vi "Find Workspace.vi"(6 "Pickup_Test_Number":dbl, 7 "Database Entry in":refnum<class "Database Entry.lvclass">, 8 "Error In":errorcluster, 9 "Assembly Type":string, 10 "Control In":T2={"I-O.lvclass"=refnum, "Gantry"=refnum, "Dispenser"="COM1"}, 11 "Workspace In":refnum<class "Fixture.lvclass">) -> (0 "Error Out":errorcluster, 1 "Workspace Out":T1, 2 "Control Out":T2={"I-O.lvclass"=refnum, "Gantry"=refnum, "Dispenser"="COM1"}, 3 "Workspace Out":refnum<class "Fixture.lvclass">, 5 "Database Entry out":refnum<class "Database Entry.lvclass">)   [LabVIEW 2021, in "Fixture.lvclass"]
uses:
  Fixture.lvclass
  Controller/Controllers.ctl
  Controller/I-O/I-O.lvclass
  C:/Program Files (x86)/Aerotech/A3200/LabVIEW/2010/Bin/Aerotech.A3200.dll
  Program Files (x86)/Aerotech/A3200/LabVIEW/2010/Bin/Aerotech.A3200.dll
  Workspace.ctl
  Assembly/Database Entry/Database Entry.lvclass
  Fixture.lvclass/Fixture.ctl
  Controller/Controller.lvclass
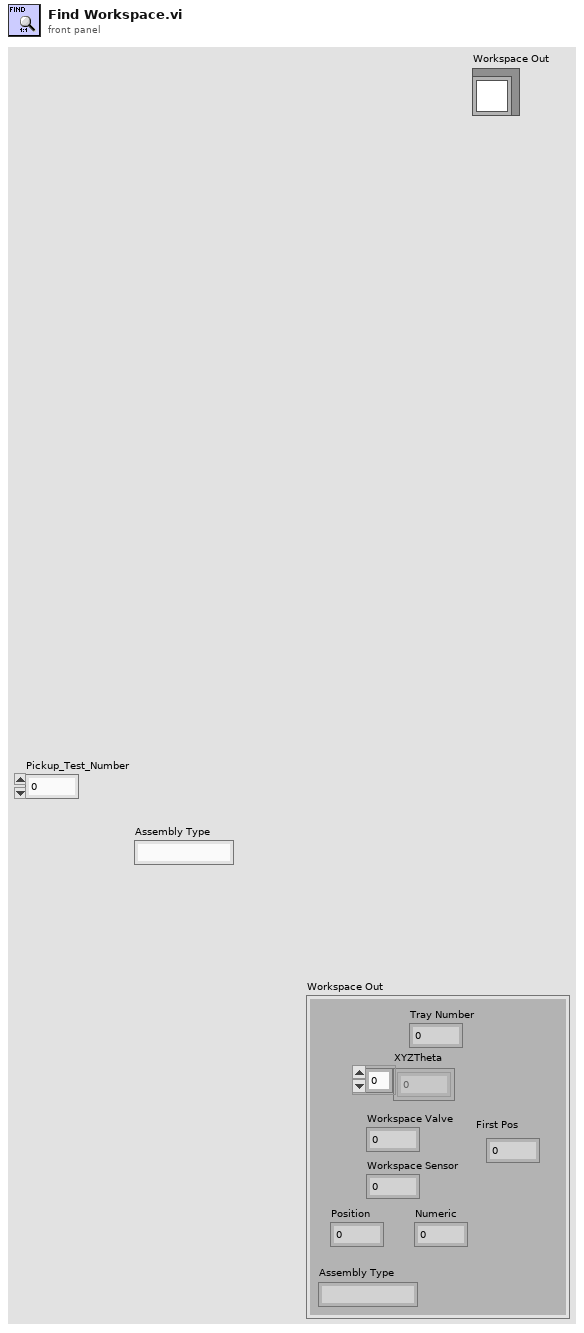
[diagram p1: front panel]
types:
  T1 = typedef "Fixture.lvclass/Workspace.ctl" = cluster{"XYZTheta":dbl[], "Workspace Valve":i32, "Workspace Sensor":i32, "Tray Number":i32, "Position":i32, "Assembly Type":string, "Numeric":dbl, "First Pos":i32}
  T2 = typedef "Controller.lvclass/Controllers.ctl" = cluster{"I-O.lvclass":refnum<class "I-O.lvclass">, "Gantry":refnum<k24>, "Dispenser":refnum<visa-resource-name>}
  T3 = typedef "I-O.lvclass/Pin Map.ctl" = cluster{"Region Valves":i32[], "Extra Valves":dbl[][][], "Tool Primary Valve":i32, "Tool Secondary Valve":i32, "Region Sensors":i32[], "Extra Sensors":dbl[][][], "Tool Primary Sensor":dbl, "Tool Secondary Sensor":dbl, "Compression Sensor":dbl, "5V":i32, "Dispenser Sensor":dbl, "Light Curtain":i32}
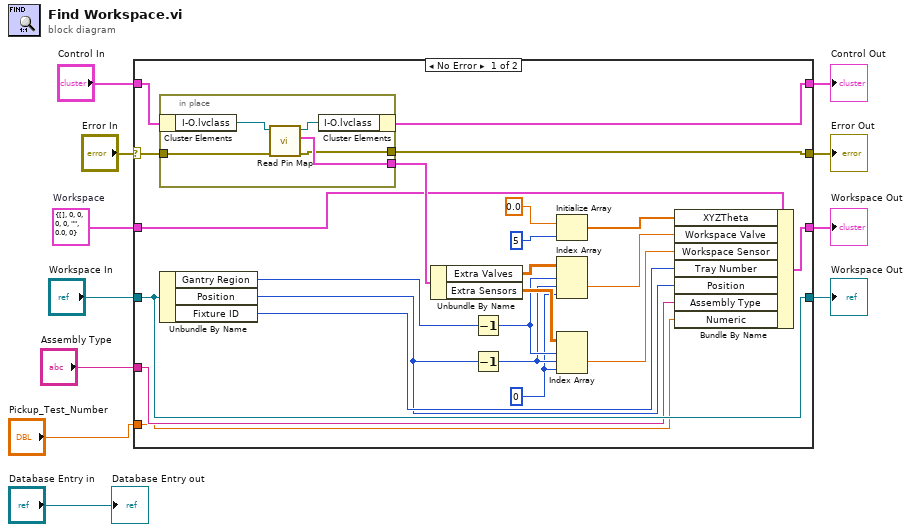
[diagram p0: block diagram]
diagram:
  w7 = T1 {"XYZTheta"=[], "Workspace Valve"=0, "Workspace Sensor"=0, "Tray Number"=0, "Position"=0, "Assembly Type"="", "Numeric"=0.0, "First Pos"=0}  # Workspace
  n1 = case shown="No Error" "Error In" {
    selector: "Error In" -> [w13 w43]
    tunnel: [w12 w43] -> w10
    tunnel: [w30 w42] -> w8
    tunnel: "Workspace In" -> [w30 w42]
    tunnel: w7 -> [w22 w41]
    tunnel: [w24 w41] -> w6
    tunnel: "Control In" -> [w34 w40]
    tunnel: [w33 w40] -> w4
    tunnel: "Assembly Type" -> [w15 _]
    tunnel: "Pickup_Test_Number" -> [w14 _]
    frame No Error {
      w18 = 0
      n2 = in-place {
        in-place-border: [w37] -> w29
        in-place-border: w13 -> [w36]
        in-place-border: [w35] -> w12
        n3 = in-place-cluster #1(w34) -> ("I-O.lvclass"=w39:refnum<class "I-O.lvclass">)
        n4 = call-dynamic "Read Pin Map.vi"("error in (no error)"=w36, "I-O in"=w39) -> ("error out"=w35:errorcluster, "Pin Map 2"=w37:T3, "I-O out"=w38:refnum<class "I-O.lvclass">)  [unwired: 7 in]
        n5 = in-place-cluster #1("I-O.lvclass"=w38) -> (w33:T2)
      }
      n6 = Unbundle By Name(w30) -> ("Gantry Region"=w21:i32, "Position"=w16:i32, "Fixture ID"=w17:i32)
      n7 = Unbundle By Name(w29) -> ("Extra Valves"=w28:dbl[][][], "Extra Sensors"=w27:dbl[][][])
      n8 = Decrement(x=w21) -> (x-1=w20:i32)
      n9 = Decrement(x=w16) -> (x-1=w19:i32)
      n10 = Initialize Array "Initialize Array"(0.0 ("element"), 5 ("dimension size")) -> (w23:dbl[])
      n11 = Index Array(array=w28, index (dim 0)=w20, index (dim 1)=w19, index (dim 2)=w18) -> (element=w26:dbl)
      n12 = Index Array "Index Array"(array=w27, index (dim 0)=w20, index (dim 1)=w19, index (dim 2)=w18) -> (element=w25:dbl)
      n13 = Bundle By Name(cluster=w22, "XYZTheta"=w23, "Workspace Valve"=w26, "Workspace Sensor"=w25, "Tray Number"=w17, "Position"=w16, "Assembly Type"=w15, "Numeric"=w14) -> (w24:T1)
    }
    frame Error {
    }
  }
  "Error Out" <- w10
  "Workspace Out" <- w8
  "Control Out" <- w4
  "Workspace Out" <- w6
  "Database Entry out" <- "Database Entry in"
